vi "__uintMaxMin.vi"(10 "Uint2 in":u8[](array[numeric])=[0], 11 "Uint1 in":u8[](array[numeric])=[0]) -> (0 "Timing":u32, 2 "Min":u8[](array[numeric]), 3 "Max":u8[](array[numeric]))   [LabVIEW 2011, in "UintClass.lvclass"]
uses:
  UintClass.lvclass
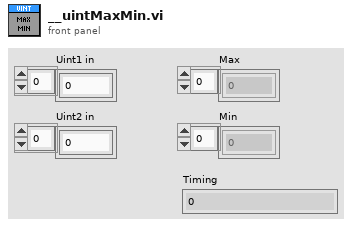
[diagram p1: front panel]
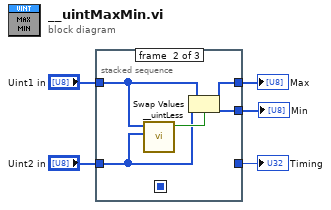
[diagram p0: block diagram]
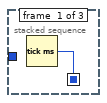
[diagram p2: hidden frame]
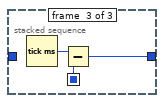
[diagram p3: hidden frame]
diagram:
  n1 = stacked-sequence {
    seq-local: [w6 _ _] -> [_ _ w13]
    tunnel: "Uint1 in" -> [_ w10 _]
    tunnel: "Uint2 in" -> [_ w9 _]
    tunnel: [_ w8 _] -> w3
    tunnel: [_ _ w12] -> w2
    tunnel: [_ w7 _] -> w1
    frame #0 {
      n2 = Tick Count (ms)() -> (millisecond timer value=w6:u32)
    }
    frame #1 {
      n3 = call "__uintLess.vi"("Uint2 in"=w9, "Uint1 in"=w10) -> ("Uint1 < Uint2"=w11:bool)  [unwired: 8 in, 1 out]
      n4 = Swap Values(12:w10, 13:w11, 14:w9) -> (1:w8:u8[], 3:w7:u8[])
    }
    frame #2 {
      n5 = Tick Count (ms)() -> (millisecond timer value=w14:u32)
      n6 = Subtract(x=w14, y=w13) -> (x-y=w12:u32)
    }
  }
  "Max" <- w3
  "Timing" <- w2
  "Min" <- w1
